vi "FormatToKeyValuePair.vi"(9 "Escape Value string?":bool=TRUE, 10 "Value":string, 11 "Key":string) -> (3 "Formatted string":string)   [LabVIEW 2017, in "JsonFormatter.lvlib"]
uses:
  JsonFormatter.lvlib
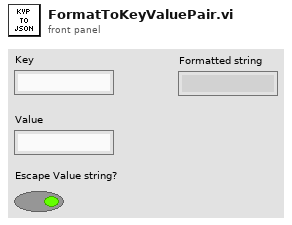
[diagram p1: front panel]
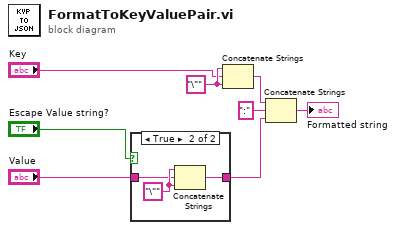
[diagram p0: block diagram]
diagram:
  w8 = "\"" ("string")
  n1 = case shown="True" "Escape Value string?" {
    tunnel: "Value" -> [w9 w11]
    tunnel: [w9 w10] -> w3
    frame False {
    }
    frame True {
      w12 = "\"" ("string")
      n2 = Concatenate Strings(w12, w11, w12) -> (w10:string)
    }
  }
  n3 = Concatenate Strings(w8, "Key", w8) -> (w4:string)
  n4 = Concatenate Strings(w4, ":" ("string"), w3) -> (→"Formatted string":string)
